vi "TPM with correction version 10-3-compare-1 scale factor_descan_20180323.vi"() -> ()   [LabVIEW 2012]
uses:
  <vilib>/_Imagine Optic/VIs drivers/Data Haso/Wavefront parameters.ctl
  Program Files/Imagine Optic/Casao LabVIEW SDK/Casao/Casao/Loop prefs.ctl
  <vilib>/_Imagine Optic/VIs drivers/Data Haso/DataHaso.ctl
  <vilib>/Utility/file.llb/Read From Spreadsheet File (DBL).vi
  <vilib>/Utility/file.llb/Write To Spreadsheet File (DBL).vi
panel:
  in  "Descan  Rescan":bool
  in  "Camera              WF sensor":bool
  in  "Scale factor":dbl=1.0
  out "output path":path
  out "Model Coefficients (µm) after":sgl[](array[numeric])
  out "Model Coefficients (µm) before":sgl[](array[numeric])
  in  "stop":bool
  out "Slice now":dbl
  in  "Iteration #":u16(ring)=1 items=["1"=1, "2"=2, "3"=3, "4"=4, "5"=5]
  in  "AoExp Time":dbl(ring)=0.5 items=["0.2s"=0.2, "0.5s"=0.5, "1.0s"=1.0, "1.5s"=1.5]
  out "after correction":T1
  in  "Filter y tilt":bool=TRUE
  in  "Filter x tilt":bool=TRUE
  in  "Curvature filter":bool=TRUE
  out "PV":dbl
  out "RMS":dbl
  in  "Matrix path":path=path "F:/Min_Data/20180327_conf_calibration/CM32.aomc"
  in  "Offset path":path=path "F:/Min_Data/100nm bead correction.dat"
  out "Camera image":u32[][](graph)
  out "RMS":dbl
  out "PV":dbl
  out "before correction":T1
  in  "Curvature filter":bool=TRUE
  in  "Filter y tilt":bool=TRUE
  in  "Filter x tilt":bool=TRUE
  out "after correction":dbl[][](graph) caption="Wavefront"
  out "before correction":dbl[][](graph) caption="Wavefront"
  in  "ImExp Time (s)":dbl(ring)=0.5 items=["0.2"=0.2, "0.5"=0.5, "1.0"=1.0, "4.0"=4.0, "8.0"=8.0]
  in  "Step size(um)":dbl
  in  "Laser Power%(0-100)":dbl=50.0
  in  "Slices #":dbl=1.0
  in  "Average Frame #":dbl=10.0
  in  "Correction":bool
  # "OFF"
  # "ON"
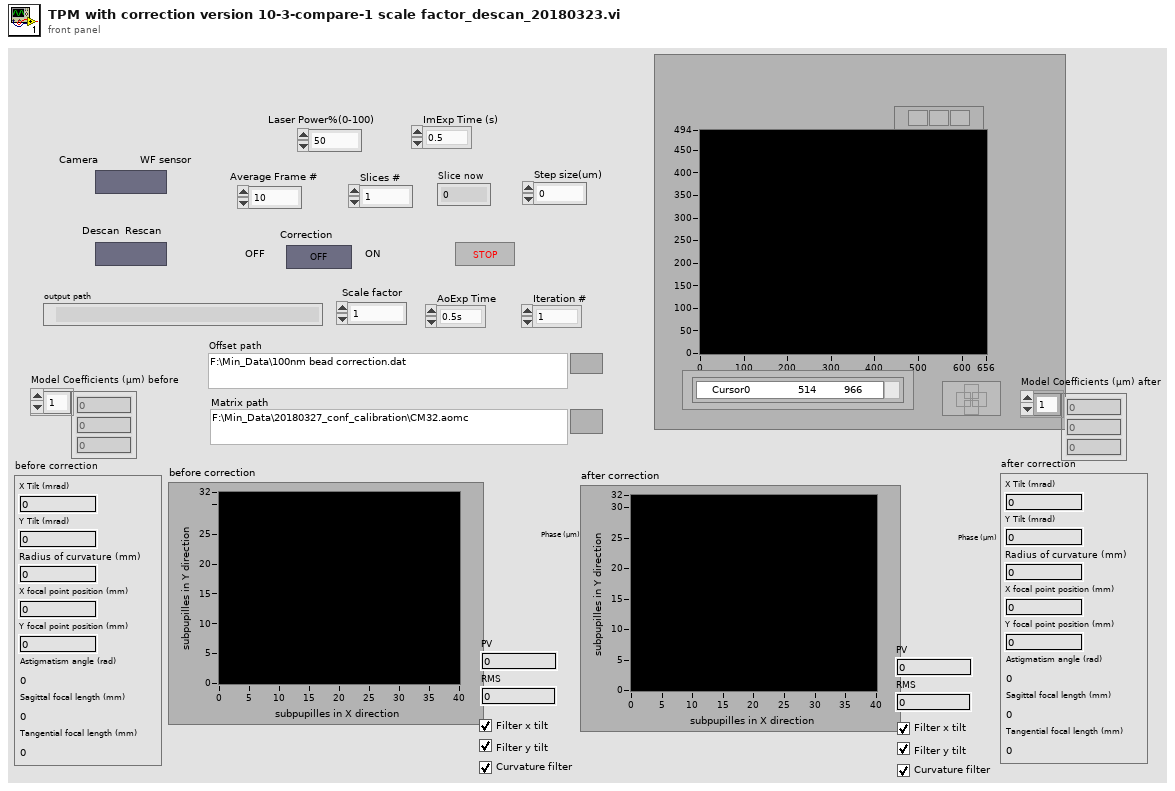
[diagram p1: front panel]
types:
  T1 = typedef "Wavefront parameters.ctl" = cluster{"X Tilt (mrad)":sgl, "Y Tilt (mrad)":sgl, "Radius of curvature (mm)":sgl, "X focal point position (mm)":sgl, "Y focal point position (mm)":sgl, "Astigmatism angle (rad)":sgl, "Sagittal focal length (mm)":sgl, "Tangential focal length (mm)":sgl}
  T2 = typedef "Loop prefs.ctl" = cluster{"Filter tilt on measurement (closed loop)":bool, "Correction gain (closed loop)":sgl, "Limit of subapertures off in CGP (%)":sgl, "Limit of saturated actuators (%)":sgl}
  T3 = cluster{"Filtre tilt X":bool, "Filtre tilt Y":bool, "Filtre courbure":bool}
  T4 = typedef "DataHaso.ctl" = i32
  T5 = cluster{"Measurement":T4, "Target":T4, "Manual target":T4}
  T6 = cluster{"Target for tilt":T4, "Target for focus":T4, "Target for all other aberrations":T4}
  T7 = typedef "Camera.ctl" = i32
  T8 = typedef "PhaseModul.ctl" = i32
  T9 = typedef "Haso.ctl" = i32
  T10 = typedef "Casao.ctl" = i32
  T11 = typedef "Image Compat.ctl" = cluster{"Signed/unsigned":bool, "Number of bits":T12, "Internal object id":i32, "Internal data id":i32}
  T12 = typedef "Data alignment enum.ctl" = enum16{"8", "16", "32"}
  T13 = typedef "Reconstruction prefs.ctl" = cluster{"Reconstruction type":enum16{"Modal", "Zonal"}, "Polynomial type":enum16{"Zernike", "Legendre"}, "Modal reconstruction prefs":T14, "Zonal reconstruction prefs":T17}
  T14 = typedef "Modal reconstruction prefs.ctl" = cluster{"Number of coefficients":u32, "Filtered coefficients":u32[], "RMS Zernike normalization":bool, "Matrix inversion method":u16, "Add zonal residual to modal fit ":bool, "Detection prefs":T15}
  T15 = typedef "PupilDetectionPrefs.ctl" = cluster{"Automatic pupil detection":bool, "Central occultation pupil":bool, "Semi-automatic pupil detection (find radius)":bool, "Semi-automatic pupil detection (find center)":bool, "Automatic pupil detection mode":enum16{"Contained", "Containing"}, "Start coordinates":cluster{"Pupil center (Zernike)":T16, "Pupil radius (Zernike)":sgl, "Pupil center (Legendre)":T16, "Pupil halfsize (Legendre)":T16}}
  T16 = typedef "Point2Df.ctl" = cluster{"X":sgl, "Y":sgl}
  T17 = typedef "Zonal reconstruction prefs.ctl" = cluster{"Number of weak iterations":u16, "Number of max iterations":u32, "Residual limit":sgl}
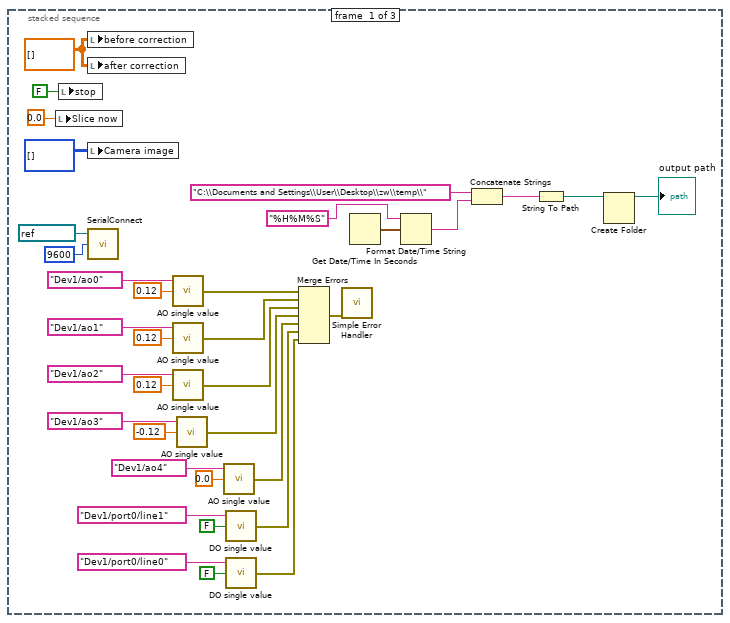
[diagram p2: hidden frame]
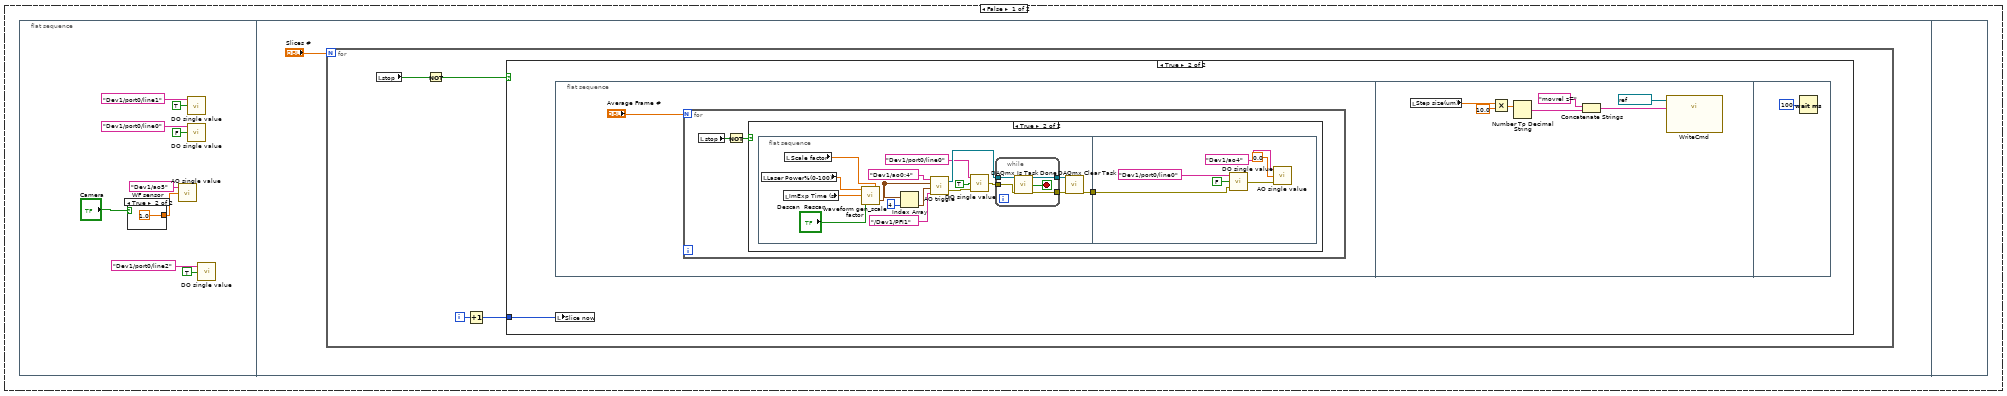
[diagram p3: hidden frame]
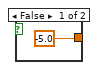
[diagram p4: hidden frame]
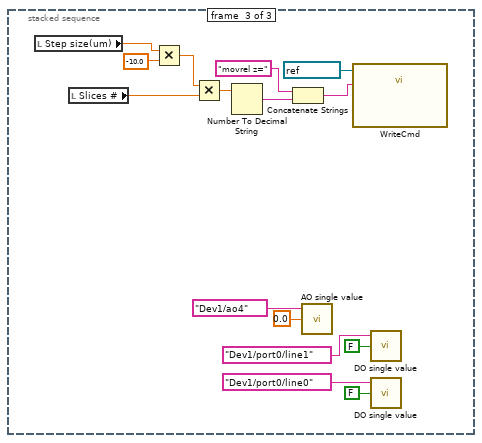
[diagram p12: hidden frame]
diagram:
  n1 = stacked-sequence {
    frame #0 {
      w34 = dbl[][] [] ("before correction")
      n2 = local write "Slice now"(0.0 ("Slice now")) -> ()
      n3 = local write "stop"(FALSE ("stop")) -> ()
      n4 = local write "before correction"(w34) -> ()
      n5 = local write "after correction"(w34) -> ()
      n6 = local write "Camera image"(u32[][] [] ("Camera image")) -> ()
      n7 = call "SerialConnect.vi"("baud rate (9600)"=u32 9600, "VISA resource name"=refnum<visa-resource-name> "COM1") -> ()  [unwired: 1 in, 3 out]
      n8 = call "AO single value.vi"("data"=0.12, "physical channels"=tag "Dev1/ao0") -> ("error out"=w17:errorcluster)  [unwired: 1 in]
      n9 = call "AO single value.vi"("data"=0.12, "physical channels"=tag "Dev1/ao1") -> ("error out"=w16:errorcluster)  [unwired: 1 in]
      n10 = call "AO single value.vi"("data"=0.12, "physical channels"=tag "Dev1/ao2") -> ("error out"=w15:errorcluster)  [unwired: 1 in]
      n11 = call "AO single value.vi"("data"=-0.12, "physical channels"=tag "Dev1/ao3") -> ("error out"=w14:errorcluster)  [unwired: 1 in]
      n12 = call "AO single value.vi"("data"=0.0, "physical channels"=tag "Dev1/ao4") -> ("error out"=w13:errorcluster)  [unwired: 1 in]
      n13 = call "DO single value.vi"("data"=FALSE, "lines"=tag "Dev1/port0/line1") -> ("error out"=w12:errorcluster)  [unwired: 1 in]
      n14 = call "DO single value.vi"("data"=FALSE, "lines"=tag "Dev1/port0/line0") -> ("error out"=w10:errorcluster)  [unwired: 1 in]
      n15 = Merge Errors(w17, w16, w15, w14, w13, w12, w10) -> (w11:errorcluster)
      n16 = call <vilib>:"Simple Error Handler.vi"("error in (no error)"=w11) -> ()  [unwired: 4 in, 5 out]
      n17 = Get Date/Time In Seconds() -> (seconds since 1Jan1904=w7:timestamp)
      n18 = Format Date/Time String(time format string (%c)="%H%M%S", seconds (now)=w7) -> (date/time string=w4:string)  [unwired: 1 in]
      n19 = Concatenate Strings("C:\\Documents and Settings\\User\\Desktop\\zw\\temp\\" ("string"), w4) -> (w3:string)
      n20 = String To Path(string=w3) -> (path=w2:path)
      n21 = Create Folder(path (use dialog)=w2) -> (created path=→"output path":path)  [unwired: 2 in, 2 out]
    }
    frame #1 {
      n22 = case shown="True" "Correction" {
        frame False {
          n23 = flat-sequence {
            frame #0 {
              n24 = case shown="True" "Camera              WF sensor" {
                tunnel: [-5.0 ("data") 1.0 ("data")] -> w40
                frame False {
                }
                frame True {
                }
              }
              n25 = call "AO single value.vi"("data"=w40, "physical channels"=tag "Dev1/ao5") -> ()  [unwired: 1 in, 1 out]
              n26 = call "DO single value.vi"("data"=TRUE, "lines"=tag "Dev1/port0/line1") -> ()  [unwired: 1 in, 1 out]
              n27 = call "DO single value.vi"("data"=FALSE, "lines"=tag "Dev1/port0/line0") -> ()  [unwired: 1 in, 1 out]
              n28 = call "DO single value.vi"("data"=TRUE, "lines"=tag "Dev1/port0/line2") -> ()  [unwired: 1 in, 1 out]
            }
            frame #1 {
              n29 = for {
                N: "Slices #" -> [_]
                i -> [w52]
                n30 = local read "stop"() -> (w50:bool)
                n31 = Not(x=w50) -> (.not. x?=w49:bool)
                n32 = Increment(x=w52) -> (x+1=w51:i32)
                n33 = case shown="True" w49 {
                  tunnel: w51 -> [_ w53]
                  frame False {
                  }
                  frame True {
                    n34 = flat-sequence {
                      frame #0 {
                        n35 = for {
                          N: "Average Frame #" -> [_]
                          n36 = local read "stop"() -> (w55:bool)
                          n37 = Not(x=w55) -> (.not. x?=w56:bool)
                          n38 = case shown="True" w56 {
                            frame False {
                            }
                            frame True {
                              n39 = flat-sequence {
                                tunnel: [w63] -> w57
                                tunnel: w57 -> [w81]
                                frame #0 {
                                n40 = local read "Laser Power%(0-100)"() -> (w60:dbl)
                                n41 = local read "ImExp Time (s)"() -> (w61:dbl)
                                n42 = local read "Scale factor"() -> (w59:dbl)
                                n43 = call "waveform gen_scale factor.vi"("Scale factor"=w59, "Boolean"="Descan  Rescan", "Exposure Time (s)"=w61, "Laser Power%(0-100)"=w60) -> ("waveform"=w62:waveform(dbl)[])
                                n44 = Index Array(array=w62, index=4) -> (element=w71:waveform(dbl))
                                n45 = call "AO triggle.vi"("physical channels"=tag "Dev1/ao0:4", "data"=w62, "waveform"=w71, "trig source"=tag "/Dev1/PFI1") -> ("task out"=w68:refnum<k21>, "error out"=w65:errorcluster)  [unwired: 1 in]
                                n46 = call "DO single value.vi"("error in"=w65, "data"=TRUE, "lines"=tag "Dev1/port0/line0") -> ("error out"=w64:errorcluster)
                                n47 = while {
                                tunnel: [w79] -> w74
                                tunnel: [w78] -> w73
                                tunnel: w68 -> [w76]
                                tunnel: w64 -> [w75]
                                stop <- w77 stop-if-true
                                n48 = call <vilib>:"DAQmx Is Task Done.vi"("task/channels in"=w76, "error in"=w75) -> ("task out"=w79:refnum<k21>, "task done?"=w77:bool, "error out"=w78:errorcluster)  [unwired: 11 in]
                                }
                                n49 = call <vilib>:"DAQmx Clear Task.vi"("task in"=w74, "error in"=w73) -> ("error out"=w63:errorcluster)  [unwired: 13 in]
                                }
                                frame #1 {
                                n50 = call "DO single value.vi"("error in"=w81, "data"=FALSE, "lines"=tag "Dev1/port0/line0") -> ("error out"=w80:errorcluster)
                                n51 = call "AO single value.vi"("error in"=w80, "data"=0.0, "physical channels"=tag "Dev1/ao4") -> ()  [unwired: 1 out]
                                }
                              }
                            }
                          }
                        }
                      }
                      frame #1 {
                        n52 = local read "Step size(um)"() -> (w86:dbl)
                        n53 = Multiply(x=w86, y=10.0) -> (x*y=w88:dbl)
                        n54 = Number To Decimal String(number=w88) -> (decimal integer string=w91:string)  [unwired: 1 in]
                        n55 = Concatenate Strings("movrel z=", w91) -> (w90:string)
                        n56 = call "WriteCmd.vi"("Command"=w90, "VISA resource name"=refnum<visa-resource-name> "COM1") -> ()  [unwired: 1 in, 1 out]
                      }
                      frame #2 {
                        n57 = Wait (ms)(milliseconds to wait=u32 100) -> ()  [unwired: 1 out]
                      }
                    }
                    n58 = local write "Slice now"(w53) -> ()
                  }
                }
              }
            }
            frame #2 {
            }
          }
        }
        frame True {
          n59 = flat-sequence {
            tunnel: [w109] -> w101
            tunnel: [w111] -> w100
            tunnel: [w110] -> w99
            tunnel: [w109] -> w98
            tunnel: [w108] -> w97
            tunnel: [w107] -> w95
            tunnel: [w102] -> w94
            tunnel: w101 -> [w128]
            tunnel: w100 -> [w127]
            tunnel: w99 -> [w126]
            tunnel: w98 -> [w122]
            tunnel: w97 -> [w120]
            tunnel: [w125] -> w96
            tunnel: w95 -> [w124]
            tunnel: w94 -> [w118]
            tunnel: w96 -> [w654]
            frame #0 {
              n60 = call "AO single value.vi"("data"=0.0, "physical channels"=tag "Dev1/ao4") -> ()  [unwired: 1 in, 1 out]
              n61 = local read "AoExp Time"() -> (w112:dbl)
              n62 = call-poly <vilib>:"Read From Spreadsheet File.vi"("format (%.3f)"="%.8f", "file path (dialog if empty)"="Offset path") -> ("first row"=w102:dbl[])  [unwired: 5 in, 4 out]
              n63 = call "DO single value.vi"("data"=TRUE, "lines"=tag "Dev1/port0/line1") -> ()  [unwired: 1 in, 1 out]
              n64 = call "DO single value.vi"("data"=FALSE, "lines"=tag "Dev1/port0/line0") -> ()  [unwired: 1 in, 1 out]
              n65 = call "AO init.vi"("Exposure duration specified (s)"=w112, "Commands in"=w102, "Matrix path"="Matrix path") -> ("error out"=w109:errorcluster, "Camera"=w111:T7, "Mirror"=w107:T8, "Haso"=w110:T9, "Casao"=w108:T10)  [unwired: 3 in, 1 out]
            }
            frame #1 {
              n66 = local read "Slices #"() -> (w129:dbl)
              n67 = call "Casao Set Preferences.vi"("error in (no error)"=w122, "Loop preferences"=T2 {"Filter tilt on measurement (closed loop)"=FALSE, "Correction gain (closed loop)"=0.75, "Limit of subapertures off in CGP (%)"=0.0, "Limit of saturated actuators (%)"=0.0}, "Casao"=w120) -> ("error out"=w121:errorcluster, "Casao (dup)"=w119:T10)  [unwired: 3 in]
              n68 = for {
                N: w129 -> [_]
                tunnel: w128 -> [w145]
                tunnel: w127 -> [w144]
                tunnel: w126 -> [w143]
                tunnel: w121 -> [w131]
                tunnel: [w142] -> w125
                tunnel: w124 -> [w133]
                tunnel: w119 -> [w141]
                tunnel: w118 -> [w134]
                i -> [w137]
                n69 = local read "stop"() -> (w139:bool)
                n70 = call "PhaseModul apply command.vi"("error in (no error)"=w131, "Commands in"=w134, "Mirror"=w133) -> ("error out"=w130:errorcluster, "Mirror (dup)"=w132:T8)  [unwired: 2 in, 1 out]
                n71 = Increment(x=w137) -> (x+1=w140:i32)
                n72 = local write "Slice now"(w140) -> ()
                n73 = Not(x=w139) -> (.not. x?=w138:bool)
                n74 = case shown="True" w138 {
                  tunnel: w145 -> [_ w180]
                  tunnel: w144 -> [_ w179]
                  tunnel: w143 -> [_ w178]
                  tunnel: w130 -> [_ w177]
                  tunnel: [w146 w174] -> w142
                  tunnel: w132 -> [_ w176]
                  tunnel: w141 -> [w146 w175]
                  frame False {
                  }
                  frame True {
                    n75 = flat-sequence {
                      tunnel: w175 -> [w185]
                      tunnel: w176 -> [w186]
                      tunnel: w177 -> [w187]
                      tunnel: w178 -> [w188]
                      tunnel: w179 -> [w189]
                      tunnel: w180 -> [w190]
                      tunnel: [w190] -> w152
                      tunnel: [w189] -> w151
                      tunnel: [w188] -> w150
                      tunnel: [w187] -> w149
                      tunnel: [w186] -> w148
                      tunnel: [w185] -> w147
                      tunnel: [w225] -> w173
                      tunnel: [w224] -> w172
                      tunnel: [w223] -> w171
                      tunnel: [w218] -> w170
                      tunnel: [w219] -> w169
                      tunnel: [w220] -> w168
                      tunnel: w152 -> [w225]
                      tunnel: w151 -> [w224]
                      tunnel: w150 -> [w223]
                      tunnel: w149 -> [w219]
                      tunnel: w148 -> [w220]
                      tunnel: w147 -> [w218]
                      tunnel: w173 -> [w267]
                      tunnel: w172 -> [w266]
                      tunnel: w171 -> [w265]
                      tunnel: w170 -> [w264]
                      tunnel: w169 -> [w263]
                      tunnel: [w243] -> w167
                      tunnel: [w242] -> w166
                      tunnel: [w238] -> w165
                      tunnel: [w236] -> w164
                      tunnel: [w234] -> w163
                      tunnel: w168 -> [w229]
                      tunnel: [w228] -> w162
                      tunnel: [w226] -> w161
                      tunnel: w167 -> [w409]
                      tunnel: w166 -> [w408]
                      tunnel: w165 -> [w406]
                      tunnel: w164 -> [w405]
                      tunnel: w163 -> [w404]
                      tunnel: [w403] -> w160
                      tunnel: w162 -> [w402]
                      tunnel: [w401] -> w159
                      tunnel: [w400] -> w158
                      tunnel: [w399] -> w157
                      tunnel: [w398] -> w156
                      tunnel: [w397] -> w155
                      tunnel: w161 -> [w396]
                      tunnel: [w396] -> w154
                      tunnel: w160 -> [w616]
                      tunnel: [w616] -> w153
                      tunnel: w159 -> [w606]
                      tunnel: w158 -> [w605]
                      tunnel: w157 -> [w604]
                      tunnel: w156 -> [w594]
                      tunnel: w155 -> [w595]
                      tunnel: w154 -> [w593]
                      tunnel: w153 -> [w617]
                      tunnel: [w617] -> w174
                      frame #0 {
                        n76 = Wait (ms)(milliseconds to wait=u32 100) -> ()  [unwired: 1 out]
                        n77 = local read "Average Frame #"() -> (w184:dbl)
                        n78 = call "AO single value.vi"("data"=-5.0, "physical channels"=tag "Dev1/ao5") -> ()  [unwired: 1 in, 1 out]
                        n79 = for {
                          N: w184 -> [_]
                          n80 = local read "stop"() -> (w191:bool)
                          n81 = Not(x=w191) -> (.not. x?=w192:bool)
                          n82 = case shown="True" w192 {
                            frame False {
                            }
                            frame True {
                              n83 = flat-sequence {
                                frame #0 {
                                n84 = local read "Laser Power%(0-100)"() -> (w194:dbl)
                                n85 = local read "ImExp Time (s)"() -> (w195:dbl)
                                n86 = local read "Scale factor"() -> (w193:dbl)
                                n87 = call "waveform gen_scale factor.vi"("Scale factor"=w193, "Boolean"=TRUE, "Exposure Time (s)"=w195, "Laser Power%(0-100)"=w194) -> ("waveform"=w197:waveform(dbl)[])
                                n88 = Index Array(array=w197, index=4) -> (element=w205:waveform(dbl))
                                n89 = call "AO triggle.vi"("physical channels"=tag "Dev1/ao0:4", "data"=w197, "waveform"=w205, "trig source"=tag "/Dev1/PFI1") -> ("task out"=w202:refnum<k21>, "error out"=w199:errorcluster)  [unwired: 1 in]
                                n90 = call "DO single value.vi"("error in"=w199, "data"=TRUE, "lines"=tag "Dev1/port0/line0") -> ("error out"=w198:errorcluster)
                                n91 = while {
                                tunnel: [w213] -> w208
                                tunnel: [w212] -> w207
                                tunnel: w202 -> [w210]
                                tunnel: w198 -> [w209]
                                stop <- w211 stop-if-true
                                n92 = call <vilib>:"DAQmx Is Task Done.vi"("task/channels in"=w210, "error in"=w209) -> ("task out"=w213:refnum<k21>, "task done?"=w211:bool, "error out"=w212:errorcluster)  [unwired: 11 in]
                                }
                                n93 = call <vilib>:"DAQmx Clear Task.vi"("task in"=w208, "error in"=w207) -> ()  [unwired: 13 in, 1 out]
                                }
                                frame #1 {
                                n94 = call "AO single value.vi"("data"=0.0, "physical channels"=tag "Dev1/ao4") -> ()  [unwired: 1 in, 1 out]
                                n95 = call "DO single value.vi"("data"=FALSE, "lines"=tag "Dev1/port0/line0") -> ()  [unwired: 1 in, 1 out]
                                }
                              }
                            }
                          }
                        }
                      }
                      frame #1 {
                        n96 = call "AO single value.vi"("data"=1.0, "physical channels"=tag "Dev1/ao5") -> ()  [unwired: 1 in, 1 out]
                      }
                      frame #2 {
                        n97 = flat-sequence {
                          tunnel: [w276] -> w262
                          tunnel: [w275] -> w261
                          tunnel: [w274] -> w260
                          tunnel: [w273] -> w259
                          tunnel: [w272] -> w258
                          tunnel: w265 -> [w274]
                          tunnel: w266 -> [w275]
                          tunnel: w267 -> [w276]
                          tunnel: [w271] -> w257
                          tunnel: w264 -> [w271]
                          tunnel: [w270] -> w256
                          tunnel: w263 -> [w270]
                          tunnel: [w269] -> w230
                          tunnel: w229 -> [w269]
                          tunnel: w262 -> [w292]
                          tunnel: w261 -> [w293]
                          tunnel: w260 -> [w294]
                          tunnel: [w294] -> w255
                          tunnel: [w291] -> w254
                          tunnel: [w290] -> w253
                          tunnel: [w289] -> w252
                          tunnel: w259 -> [w289]
                          tunnel: [w288] -> w251
                          tunnel: w258 -> [w288]
                          tunnel: [w287] -> w250
                          tunnel: w257 -> [w287]
                          tunnel: [w286] -> w249
                          tunnel: w256 -> [w286]
                          tunnel: [w285] -> w231
                          tunnel: w230 -> [w285]
                          tunnel: w255 -> [w306]
                          tunnel: [w306] -> w246
                          tunnel: [w305] -> w247
                          tunnel: w254 -> [w305]
                          tunnel: [w304] -> w248
                          tunnel: w253 -> [w304]
                          tunnel: w252 -> [w299]
                          tunnel: w251 -> [w298]
                          tunnel: [w297] -> w245
                          tunnel: w250 -> [w297]
                          tunnel: [w296] -> w244
                          tunnel: w249 -> [w296]
                          tunnel: [w295] -> w232
                          tunnel: w231 -> [w295]
                          tunnel: w248 -> [w388]
                          tunnel: w247 -> [w348]
                          tunnel: w246 -> [w349]
                          tunnel: w245 -> [w374]
                          tunnel: w244 -> [w373]
                          tunnel: [w352] -> w241
                          tunnel: [w351] -> w240
                          tunnel: [w350] -> w239
                          tunnel: [w349] -> w237
                          tunnel: [w348] -> w235
                          tunnel: [w347] -> w233
                          tunnel: w232 -> [w346]
                          tunnel: [w346] -> w227
                          tunnel: [w320] -> w226
                          tunnel: [w394] -> w242
                          tunnel: [w395] -> w243
                          tunnel: w241 -> [w395]
                          tunnel: w240 -> [w394]
                          tunnel: w239 -> [w393]
                          tunnel: [w392] -> w238
                          tunnel: w237 -> [w392]
                          tunnel: [w391] -> w236
                          tunnel: w235 -> [w391]
                          tunnel: [w390] -> w234
                          tunnel: w233 -> [w390]
                          tunnel: [w389] -> w228
                          tunnel: w227 -> [w389]
                          frame #0 {
                            n98 = local read "Laser Power%(0-100)"() -> (w282:dbl)
                            n99 = local read "AoExp Time"() -> (w281:dbl)
                            n100 = local read "Scale factor"() -> (w268:dbl)
                            n101 = call "waveform gen_scale factor.vi"("Scale factor"=w268, "Boolean"=FALSE, "Exposure Time (s)"=w281, "Laser Power%(0-100)"=w282) -> ("waveform"=w280:waveform(dbl)[])
                            n102 = Index Array(array=w280, index=4) -> (element=w279:waveform(dbl))
                            n103 = call "AO triggle.vi"("physical channels"=tag "Dev1/ao0:4", "data"=w280, "waveform"=w279, "trig source"=tag "/Dev1/PFI1") -> ("task out"=w273:refnum<k21>, "error out"=w272:errorcluster)  [unwired: 1 in]
                          }
                          frame #1 {
                            n104 = call <vilib>:"Camera Start.vi"("error in (no error)"=w292, "camera"=w293) -> ("error out"=w290:errorcluster, "camera (dup)"=w291:T7)  [unwired: 4 in]
                          }
                          frame #2 {
                            n105 = while {
                              tunnel: [w311] -> w301
                              tunnel: [w310] -> w300
                              tunnel: w299 -> [w308]
                              tunnel: w298 -> [w307]
                              stop <- w309 stop-if-true
                              n106 = call <vilib>:"DAQmx Is Task Done.vi"("task/channels in"=w308, "error in"=w307) -> ("task out"=w311:refnum<k21>, "task done?"=w309:bool, "error out"=w310:errorcluster)  [unwired: 11 in]
                            }
                            n107 = call "DO single value.vi"("data"=TRUE, "lines"=tag "Dev1/port0/line0") -> ()  [unwired: 1 in, 1 out]
                            n108 = call <vilib>:"DAQmx Clear Task.vi"("task in"=w301, "error in"=w300) -> ()  [unwired: 13 in, 1 out]
                          }
                          frame #3 {
                            n109 = call <vilib>:"Camera Get image.vi"("error in (no error)"=w388, "camera"=w348) -> ("error out"=w370:errorcluster, "Image"=w371:T11, "camera (dup)"=w372:T7)  [unwired: 3 in]
                            n110 = call <vilib>:"Camera Stop.vi"("error in (no error)"=w370, "camera"=w372) -> ()  [unwired: 4 in, 2 out]
                            n111 = call "Image get data.vi"("error in (no error)"=w370, "Image Compat"=w371) -> ("error out"=w360:errorcluster, "Array"=w369:u32[][], "Image Compat (dup)"=w359:T11)  [unwired: 3 in]
                            n112 = call "AO single value.vi"("data"=0.0, "physical channels"=tag "Dev1/ao4") -> ()  [unwired: 1 in, 1 out]
                            n113 = local write "Camera image"(w369) -> ()
                            n114 = call <vilib>:"Haso compute slopes.vi"("error in (no error)"=w360, "Image Compat"=w359, "Haso"=w349) -> ("error out"=w318:errorcluster, "Data Haso"=w322:T4)  [unwired: 1 in, 2 out]
                            n115 = call "DO single value.vi"("data"=FALSE, "lines"=tag "Dev1/port0/line0") -> ()  [unwired: 1 in, 1 out]
                            n116 = call "DataHaso ctor copie.vi"("error in (no error)"=w318, "DataHaso"=w322) -> ("error out"=w317:errorcluster, "new DataHaso"=w320:T4, "DataHaso (dup)"=w319:T4)  [unwired: 3 in]
                            n117 = call "DataHaso get reconstruction prefs.vi"("error in (no error)"=w317, "Data Haso"=w319) -> ("error out"=w333:errorcluster, "Reconstruction Preferences"=w329:T13, "Data Haso (dup)"=w332:T4)  [unwired: 3 in]
                            n118 = Bundle By Name(cluster=w329, "Reconstruction type"=enum16{"Modal", "Zonal"}."Modal", "Polynomial type"=enum16{"Zernike", "Legendre"}."Zernike", "Modal reconstruction prefs.Number of coefficients"=u32 32) -> (w328:T13)
                            n119 = call <vilib>:"DataHaso set reconstruction prefs.vi"("error in (no error)"=w333, "Reconstruction Preferences"=w328, "Data Haso"=w332) -> ("error out"=w330:errorcluster, "Data Haso (dup)"=w331:T4)  [unwired: 3 in]
                            n120 = call "DataHaso get modal coefficients.vi"("error in (no error)"=w330, "Data Haso"=w331) -> ("error out"=w323:errorcluster, "Coefficients (µm)"=w334:sgl[], "Data Haso (dup)"=w324:T4)  [unwired: 3 in]
                            "Model Coefficients (µm) before" <- w334
                            n121 = Bundle By Name(cluster=T3 {"Filtre tilt X"=FALSE, "Filtre tilt Y"=FALSE, "Filtre courbure"=FALSE} ("Filtre"), "Filtre tilt X"="Filter x tilt", "Filtre tilt Y"="Filter y tilt", "Filtre courbure"="Curvature filter") -> (w354:T3)
                            n122 = call <vilib>:"DataHaso parameters.vi"("error in (no error)"=w323, "Data Haso"=w324) -> ("error out"=w367:errorcluster, "Parameters"=w342:T1, "Data Haso (dup)"=w368:T4)  [unwired: 3 in]
                            "before correction" <- w342
                            n123 = control-ref of="before correction"() -> (w353:refnum<vi>)
                            n124 = Cluster To Array(cluster=w342) -> (array=w343:sgl[])
                            n125 = call "DataHaso filter tilt or curvature.vi"("error in (no error)"=w367, "Filter (default: all true)"=w354, "Data Haso"=w368) -> ("error out"=w365:errorcluster, "Data Haso (dup)"=w366:T4)  [unwired: 3 in]
                            n126 = local read "Slice now"() -> (w336:dbl)
                            n127 = call "DataHaso phase.vi"("error in (no error)"=w365, "Data Haso"=w366) -> ("error out"=w363:errorcluster, "Phase (µm)"=w364:i32, "Data Haso (dup)"=w321:T4)  [unwired: 3 in]
                            n128 = Number To Decimal String(number=w336) -> (decimal integer string=w338:string)  [unwired: 1 in]
                            n129 = call "Formatter Intensity Graph.vi"("error in (no error)"=w363, "Intensity Graph"=w353, "Surface with pupil"=w364) -> ("error out"=w361:errorcluster, "Surface with pupil (dup)"=w362:i32)  [unwired: 2 in, 1 out]
                            n130 = call <vilib>:"Surface with pupil get stats.vi"("error in (no error)"=w361, "Surface Avec Pupille"=w362) -> ("error out"=w347:errorcluster, "PV"=w345:sgl, "RMS"=w344:dbl)  [unwired: 2 in, 1 out]
                            "PV" <- w345
                            "RMS" <- w344
                            n131 = local read "output path"() -> (w314:path)
                            n132 = Concatenate Strings("before_slice", w338, ".dat") -> (w313:string)
                            n133 = Build Path(base path=w314, name or relative path=w313) -> (appended path=w312:path)
                            n134 = Build Array (concatenate)(w345, w344, w343, w334) -> (w341:dbl[])
                            n135 = Merge Errors(w347, w373) -> (w383:errorcluster)
                            n136 = Bundle By Name(cluster=T6 {"Target for tilt"=0, "Target for focus"=0, "Target for all other aberrations"=0} ("References"), "Target for tilt"=w320, "Target for focus"=w320) -> (w386:T6)
                            n137 = call "DataHaso ctor copie.vi"("error in (no error)"=w383, "DataHaso"=w321) -> ("error out"=w385:errorcluster, "new DataHaso"=w384:T4)  [unwired: 3 in, 1 out]
                            n138 = call-poly <vilib>:"Write To Spreadsheet File.vi"("transpose? (no:F)"=TRUE, "format (%.3f)"="%.6f", "1D data"=w341, "file path (dialog if empty)"=w312) -> ()  [unwired: 4 in, 1 out]
                            n139 = call "Casao Compute target.vi"("error in (no error)"=w385, "Targets"=w386, "DataHaso"=w384, "Casao"=w374) -> ("error out"=w381:errorcluster, "DataHaso (dup)"=w350:T4, "Casao (dup)"=w382:T10)  [unwired: 1 out]
                            n140 = Bundle By Name(cluster=T5 {"Measurement"=0, "Target"=0, "Manual target"=0} ("Slopes"), "Measurement"=w321, "Target"=w350) -> (w380:T5)
                            n141 = call "Casao get correction commands.vi"("Casao"=w382, "Slopes"=w380, "error in (no error)"=w381) -> ("Casao (dup)"=w352:T10, "Commands"=w377:sgl[], "error out"=w378:errorcluster)  [unwired: 2 in, 2 out]
                            n142 = call "PhaseModul apply command.vi"("error in (no error)"=w378, "Commands in"=w377, "Mirror"=w346) -> ("error out"=w351:errorcluster)  [unwired: 2 in, 2 out]
                          }
                          frame #4 {
                            n143 = call "DataHaso dtor.vi"("Data Haso"=w393) -> ()  [unwired: 6 in, 1 out]
                          }
                        }
                      }
                      frame #3 {
                        n144 = for {
                          N: "Iteration #" -> [_]
                          tunnel: w409 -> [w438]
                          tunnel: w408 -> [w437]
                          tunnel: w406 -> [w436]
                          tunnel: w405 -> [w435]
                          tunnel: w404 -> [w434]
                          tunnel: [w432] -> w403
                          tunnel: w402 -> [w427]
                          tunnel: [w426] -> w401
                          tunnel: [w424] -> w400
                          tunnel: [w422] -> w399
                          tunnel: [w420] -> w398
                          tunnel: [w417] -> w397
                          tunnel: w396 -> [w416]
                          i -> [w415]
                          n145 = Increment(x=w415) -> (x+1=w414:i32)
                          n146 = flat-sequence {
                            tunnel: [w463] -> w457
                            tunnel: [w464] -> w456
                            tunnel: [w465] -> w455
                            tunnel: [w469] -> w454
                            tunnel: [w468] -> w453
                            tunnel: [w467] -> w452
                            tunnel: [w466] -> w451
                            tunnel: w438 -> [w467]
                            tunnel: w437 -> [w466]
                            tunnel: w436 -> [w465]
                            tunnel: w435 -> [w464]
                            tunnel: w434 -> [w463]
                            tunnel: [w462] -> w428
                            tunnel: w427 -> [w462]
                            tunnel: w414 -> [w460]
                            tunnel: [w459] -> w411
                            tunnel: w457 -> [w486]
                            tunnel: w456 -> [w487]
                            tunnel: w455 -> [w488]
                            tunnel: [w488] -> w450
                            tunnel: [w485] -> w449
                            tunnel: [w484] -> w448
                            tunnel: [w483] -> w447
                            tunnel: w454 -> [w483]
                            tunnel: [w482] -> w446
                            tunnel: w453 -> [w482]
                            tunnel: [w481] -> w445
                            tunnel: w452 -> [w481]
                            tunnel: [w480] -> w444
                            tunnel: w451 -> [w480]
                            tunnel: [w479] -> w429
                            tunnel: w428 -> [w479]
                            tunnel: [w478] -> w412
                            tunnel: w411 -> [w478]
                            tunnel: w450 -> [w501]
                            tunnel: [w501] -> w441
                            tunnel: [w500] -> w442
                            tunnel: w449 -> [w500]
                            tunnel: [w499] -> w443
                            tunnel: w448 -> [w499]
                            tunnel: w447 -> [w494]
                            tunnel: w446 -> [w493]
                            tunnel: [w492] -> w440
                            tunnel: w445 -> [w492]
                            tunnel: [w491] -> w439
                            tunnel: w444 -> [w491]
                            tunnel: [w490] -> w430
                            tunnel: w429 -> [w490]
                            tunnel: [w489] -> w413
                            tunnel: w412 -> [w489]
                            tunnel: w443 -> [w569]
                            tunnel: w442 -> [w570]
                            tunnel: w441 -> [w571]
                            tunnel: w440 -> [w556]
                            tunnel: w439 -> [w555]
                            tunnel: [w535] -> w433
                            tunnel: [w534] -> w431
                            tunnel: w430 -> [w514]
                            tunnel: [w530] -> w425
                            tunnel: [w529] -> w423
                            tunnel: [w528] -> w421
                            tunnel: [w527] -> w419
                            tunnel: [w516] -> w418
                            tunnel: w416 -> [w513]
                            tunnel: w413 -> [w510]
                            tunnel: [w507] -> w410
                            tunnel: w433 -> [w583]
                            tunnel: [w582] -> w432
                            tunnel: w431 -> [w582]
                            tunnel: [w581] -> w426
                            tunnel: w425 -> [w581]
                            tunnel: [w580] -> w424
                            tunnel: w423 -> [w580]
                            tunnel: [w579] -> w422
                            tunnel: w421 -> [w579]
                            tunnel: [w575] -> w420
                            tunnel: w419 -> [w576]
                            tunnel: w418 -> [w578]
                            tunnel: [w578] -> w417
                            tunnel: w410 -> [w577]
                            frame #0 {
                              n147 = local read "Laser Power%(0-100)"() -> (w475:dbl)
                              n148 = local read "AoExp Time"() -> (w474:dbl)
                              n149 = local read "Scale factor"() -> (w458:dbl)
                              n150 = call "waveform gen_scale factor.vi"("Scale factor"=w458, "Boolean"=FALSE, "Exposure Time (s)"=w474, "Laser Power%(0-100)"=w475) -> ("waveform"=w473:waveform(dbl)[])
                              n151 = local read "Iteration #"() -> (w461:u16)
                              n152 = Index Array(array=w473, index=4) -> (element=w472:waveform(dbl))
                              n153 = Less?(x=w461, y=w460) -> (x < y?=w459:bool)
                              n154 = call "AO triggle.vi"("physical channels"=tag "Dev1/ao0:4", "data"=w473, "waveform"=w472, "trig source"=tag "/Dev1/PFI1") -> ("task out"=w469:refnum<k21>, "error out"=w468:errorcluster)  [unwired: 1 in]
                            }
                            frame #1 {
                              n155 = call <vilib>:"Camera Start.vi"("error in (no error)"=w486, "camera"=w487) -> ("error out"=w484:errorcluster, "camera (dup)"=w485:T7)  [unwired: 4 in]
                            }
                            frame #2 {
                              n156 = while {
                                tunnel: [w506] -> w496
                                tunnel: [w505] -> w495
                                tunnel: w494 -> [w503]
                                tunnel: w493 -> [w502]
                                stop <- w504 stop-if-true
                                n157 = call <vilib>:"DAQmx Is Task Done.vi"("task/channels in"=w503, "error in"=w502) -> ("task out"=w506:refnum<k21>, "task done?"=w504:bool, "error out"=w505:errorcluster)  [unwired: 11 in]
                              }
                              n158 = call "DO single value.vi"("data"=TRUE, "lines"=tag "Dev1/port0/line0") -> ()  [unwired: 1 in, 1 out]
                              n159 = call <vilib>:"DAQmx Clear Task.vi"("task in"=w496, "error in"=w495) -> ()  [unwired: 13 in, 1 out]
                            }
                            frame #3 {
                              n160 = call <vilib>:"Camera Get image.vi"("error in (no error)"=w569, "camera"=w570) -> ("error out"=w552:errorcluster, "Image"=w553:T11, "camera (dup)"=w554:T7)  [unwired: 3 in]
                              n161 = call <vilib>:"Camera Stop.vi"("error in (no error)"=w552, "camera"=w554) -> ()  [unwired: 4 in, 2 out]
                              n162 = call "Image get data.vi"("error in (no error)"=w552, "Image Compat"=w553) -> ("error out"=w542:errorcluster, "Array"=w551:u32[][], "Image Compat (dup)"=w541:T11)  [unwired: 3 in]
                              n163 = call "AO single value.vi"("data"=0.0, "physical channels"=tag "Dev1/ao4") -> ()  [unwired: 1 in, 1 out]
                              n164 = local write "Camera image"(w551) -> ()
                              n165 = call <vilib>:"Haso compute slopes.vi"("error in (no error)"=w542, "Image Compat"=w541, "Haso"=w571) -> ("error out"=w519:errorcluster, "Data Haso"=w518:T4)  [unwired: 1 in, 2 out]
                              n166 = call "DO single value.vi"("data"=FALSE, "lines"=tag "Dev1/port0/line0") -> ()  [unwired: 1 in, 1 out]
                              n167 = call "DataHaso get reconstruction prefs.vi"("error in (no error)"=w519, "Data Haso"=w518) -> ("error out"=w525:errorcluster, "Reconstruction Preferences"=w524:T13, "Data Haso (dup)"=w526:T4)  [unwired: 3 in]
                              n168 = Bundle By Name(cluster=w524, "Reconstruction type"=enum16{"Modal", "Zonal"}."Modal", "Polynomial type"=enum16{"Zernike", "Legendre"}."Zernike", "Modal reconstruction prefs.Number of coefficients"=u32 32) -> (w523:T13)
                              n169 = call <vilib>:"DataHaso set reconstruction prefs.vi"("error in (no error)"=w525, "Reconstruction Preferences"=w523, "Data Haso"=w526) -> ("error out"=w511:errorcluster, "Data Haso (dup)"=w512:T4)  [unwired: 3 in]
                              n170 = call "DataHaso get modal coefficients.vi"("error in (no error)"=w511, "Data Haso"=w512) -> ("error out"=w517:errorcluster, "Coefficients (µm)"=w516:sgl[], "Data Haso (dup)"=w515:T4)  [unwired: 3 in]
                              "Model Coefficients (µm) after" <- w516
                              n171 = Bundle By Name(cluster=T3 {"Filtre tilt X"=FALSE, "Filtre tilt Y"=FALSE, "Filtre courbure"=FALSE} ("Filtre"), "Filtre tilt X"="Filter x tilt", "Filtre tilt Y"="Filter y tilt", "Filtre courbure"="Curvature filter") -> (w539:T3)
                              n172 = call <vilib>:"DataHaso parameters.vi"("error in (no error)"=w517, "Data Haso"=w515) -> ("error out"=w549:errorcluster, "Parameters"=w528:T1, "Data Haso (dup)"=w550:T4)  [unwired: 3 in]
                              "after correction" <- w528
                              n173 = control-ref of="after correction"() -> (w533:refnum<vi>)
                              n174 = call "DataHaso filter tilt or curvature.vi"("error in (no error)"=w549, "Filter (default: all true)"=w539, "Data Haso"=w550) -> ("error out"=w547:errorcluster, "Data Haso (dup)"=w548:T4)  [unwired: 3 in]
                              n175 = call "DataHaso phase.vi"("error in (no error)"=w547, "Data Haso"=w548) -> ("error out"=w545:errorcluster, "Phase (µm)"=w546:i32, "Data Haso (dup)"=w532:T4)  [unwired: 3 in]
                              n176 = call "Formatter Intensity Graph.vi"("error in (no error)"=w545, "Intensity Graph"=w533, "Surface with pupil"=w546) -> ("error out"=w543:errorcluster, "Surface with pupil (dup)"=w544:i32)  [unwired: 2 in, 1 out]
                              n177 = call <vilib>:"Surface with pupil get stats.vi"("error in (no error)"=w543, "Surface Avec Pupille"=w544) -> ("error out"=w564:errorcluster, "PV"=w529:sgl, "RMS"=w530:dbl)  [unwired: 2 in, 1 out]
                              "RMS" <- w530
                              "PV" <- w529
                              n178 = Merge Errors(w564, w555) -> (w563:errorcluster)
                              n179 = Bundle By Name(cluster=T6 {"Target for tilt"=0, "Target for focus"=0, "Target for all other aberrations"=0} ("References"), "Target for tilt"=w513, "Target for focus"=w513) -> (w567:T6)
                              n180 = call "DataHaso ctor copie.vi"("error in (no error)"=w563, "DataHaso"=w532) -> ("error out"=w566:errorcluster, "new DataHaso"=w565:T4, "DataHaso (dup)"=w531:T4)  [unwired: 3 in]
                              n181 = call "Casao Compute target.vi"("error in (no error)"=w566, "Targets"=w567, "DataHaso"=w565, "Casao"=w556) -> ("error out"=w561:errorcluster, "DataHaso (dup)"=w535:T4, "Casao (dup)"=w562:T10)  [unwired: 1 out]
                              n182 = Bundle By Name(cluster=T5 {"Measurement"=0, "Target"=0, "Manual target"=0} ("Slopes"), "Measurement"=w531, "Target"=w535) -> (w560:T5)
                              n183 = call "Casao get correction commands.vi"("Casao"=w562, "Slopes"=w560, "error in (no error)"=w561) -> ("Casao (dup)"=w534:T10, "Commands"=w527:sgl[], "error out"=w507:errorcluster)  [unwired: 2 in, 2 out]
                              n184 = case shown="True" w510 {
                                tunnel: w507 -> [_ w574]
                                tunnel: w527 -> [_ w573]
                                tunnel: w514 -> [_ w572]
                                frame False {
                                }
                                frame True {
                                n185 = call "PhaseModul apply command.vi"("error in (no error)"=w574, "Commands in"=w573, "Mirror"=w572) -> ()  [unwired: 2 in, 3 out]
                                }
                              }
                            }
                            frame #4 {
                              n186 = call "DataHaso dtor.vi"("Data Haso"=w583) -> ()  [unwired: 6 in, 1 out]
                              n187 = case shown="Error" w577 {
                                tunnel: w576 -> [w584 _]
                                tunnel: [w584 w585] -> w575
                                frame No Error {
                                }
                                frame Error {
                                n188 = Initialize Array(0.0 ("element"), 52 ("dimension size")) -> (w585:dbl[])
                                }
                              }
                            }
                          }
                        }
                      }
                      frame #4 {
                        n189 = call "DataHaso dtor.vi"("Data Haso"=w593) -> ()  [unwired: 6 in, 1 out]
                        n190 = local read "Slice now"() -> (w598:dbl)
                        n191 = Cluster To Array(cluster=w604) -> (array=w603:sgl[])
                        n192 = Build Array (concatenate)(w605, w606, w603, w595) -> (w611:dbl[])
                        n193 = Number To Decimal String(number=w598) -> (decimal integer string=w608:string)  [unwired: 1 in]
                        n194 = Number To Decimal String(number=w598) -> (decimal integer string=w600:string)  [unwired: 1 in]
                        n195 = call "AO single value.vi"("data"=0.0, "physical channels"=tag "Dev1/ao4") -> ()  [unwired: 1 in, 1 out]
                        n196 = call "AO single value.vi"("data"=-5.0, "physical channels"=tag "Dev1/ao5") -> ()  [unwired: 1 in, 1 out]
                        n197 = local read "output path"() -> (w592:path)
                        n198 = Concatenate Strings("afterC_slice", w608, ".dat") -> (w591:string)
                        n199 = Concatenate Strings("command", w600, ".dat") -> (w589:string)
                        n200 = Build Path(base path=w592, name or relative path=w591) -> (appended path=w590:path)
                        n201 = Build Path(base path=w592, name or relative path=w589) -> (appended path=w588:path)
                        n202 = call-poly <vilib>:"Write To Spreadsheet File.vi"("transpose? (no:F)"=TRUE, "format (%.3f)"="%.6f", "1D data"=w611, "file path (dialog if empty)"=w590) -> ()  [unwired: 4 in, 1 out]
                        n203 = call-poly <vilib>:"Write To Spreadsheet File.vi"("transpose? (no:F)"=TRUE, "format (%.3f)"="%.6f", "1D data"=w594, "file path (dialog if empty)"=w588) -> ()  [unwired: 4 in, 1 out]
                      }
                      frame #5 {
                        n204 = local read "Average Frame #"() -> (w618:dbl)
                        n205 = for {
                          N: w618 -> [_]
                          n206 = local read "stop"() -> (w619:bool)
                          n207 = Not(x=w619) -> (.not. x?=w620:bool)
                          n208 = case shown="True" w620 {
                            frame False {
                            }
                            frame True {
                              n209 = flat-sequence {
                                frame #0 {
                                n210 = local read "Laser Power%(0-100)"() -> (w622:dbl)
                                n211 = local read "Scale factor"() -> (w621:dbl)
                                n212 = local read "ImExp Time (s)"() -> (w623:dbl)
                                n213 = call "waveform gen_scale factor.vi"("Scale factor"=w621, "Boolean"=TRUE, "Exposure Time (s)"=w623, "Laser Power%(0-100)"=w622) -> ("waveform"=w625:waveform(dbl)[])
                                n214 = Index Array(array=w625, index=4) -> (element=w633:waveform(dbl))
                                n215 = call "AO triggle.vi"("physical channels"=tag "Dev1/ao0:4", "data"=w625, "waveform"=w633, "trig source"=tag "/Dev1/PFI1") -> ("task out"=w630:refnum<k21>, "error out"=w627:errorcluster)  [unwired: 1 in]
                                n216 = call "DO single value.vi"("error in"=w627, "data"=TRUE, "lines"=tag "Dev1/port0/line0") -> ("error out"=w626:errorcluster)
                                n217 = while {
                                tunnel: [w641] -> w636
                                tunnel: [w640] -> w635
                                tunnel: w630 -> [w638]
                                tunnel: w626 -> [w637]
                                stop <- w639 stop-if-true
                                n218 = call <vilib>:"DAQmx Is Task Done.vi"("task/channels in"=w638, "error in"=w637) -> ("task out"=w641:refnum<k21>, "task done?"=w639:bool, "error out"=w640:errorcluster)  [unwired: 11 in]
                                }
                                n219 = call <vilib>:"DAQmx Clear Task.vi"("task in"=w636, "error in"=w635) -> ()  [unwired: 13 in, 1 out]
                                }
                                frame #1 {
                                n220 = call "AO single value.vi"("data"=0.0, "physical channels"=tag "Dev1/ao4") -> ()  [unwired: 1 in, 1 out]
                                n221 = call "DO single value.vi"("data"=FALSE, "lines"=tag "Dev1/port0/line0") -> ()  [unwired: 1 in, 1 out]
                                }
                              }
                            }
                          }
                        }
                      }
                      frame #6 {
                        n222 = local read "Step size(um)"() -> (w652:dbl)
                        n223 = Multiply(x=w652, y=10.0) -> (x*y=w650:dbl)
                        n224 = Number To Decimal String(number=w650) -> (decimal integer string=w647:string)  [unwired: 1 in]
                        n225 = Concatenate Strings("movrel z=", w647) -> (w648:string)
                        n226 = call "WriteCmd.vi"("Command"=w648, "VISA resource name"=refnum<visa-resource-name> "COM1") -> ()  [unwired: 1 in, 1 out]
                      }
                      frame #7 {
                        n227 = Wait (ms)(milliseconds to wait=u32 50) -> ()  [unwired: 1 out]
                      }
                    }
                  }
                }
                n228 = call "AO single value.vi"("data"=0.0, "physical channels"=tag "Dev1/ao4") -> ()  [unwired: 1 in, 1 out]
              }
            }
            frame #2 {
              n229 = call "Casao dtor.vi"("Casao"=w654) -> ()  [unwired: 6 in, 1 out]
            }
          }
        }
      }
    }
    frame #2 {
      n230 = local read "Step size(um)"() -> (w662:dbl)
      n231 = local read "Slices #"() -> (w655:dbl)
      n232 = Multiply(x=w662, y=-10.0) -> (x*y=w663:dbl)
      n233 = Multiply(x=w663, y=w655) -> (x*y=w661:dbl)
      n234 = Number To Decimal String(number=w661) -> (decimal integer string=w657:string)  [unwired: 1 in]
      n235 = Concatenate Strings("movrel z=", w657) -> (w658:string)
      n236 = call "AO single value.vi"("data"=0.0, "physical channels"=tag "Dev1/ao4") -> ()  [unwired: 1 in, 1 out]
      n237 = call "WriteCmd.vi"("Command"=w658, "VISA resource name"=refnum<visa-resource-name> "COM1") -> ()  [unwired: 1 in, 1 out]
      n238 = call "DO single value.vi"("data"=FALSE, "lines"=tag "Dev1/port0/line1") -> ()  [unwired: 1 in, 1 out]
      n239 = call "DO single value.vi"("data"=FALSE, "lines"=tag "Dev1/port0/line0") -> ()  [unwired: 1 in, 1 out]
    }
  }
